vi "WRITE CAN DATA.vi"(7 "Enum":T2=enum."GET", 11 "CAN DATA":T1[](array[typedef])) -> (3 "READ DATA OUT":T1[](array[typedef]))   [LabVIEW 2025]
uses:
  Controls/READ CAN DATA.ctl
  Controls/READ CAN CLUSTER.ctl
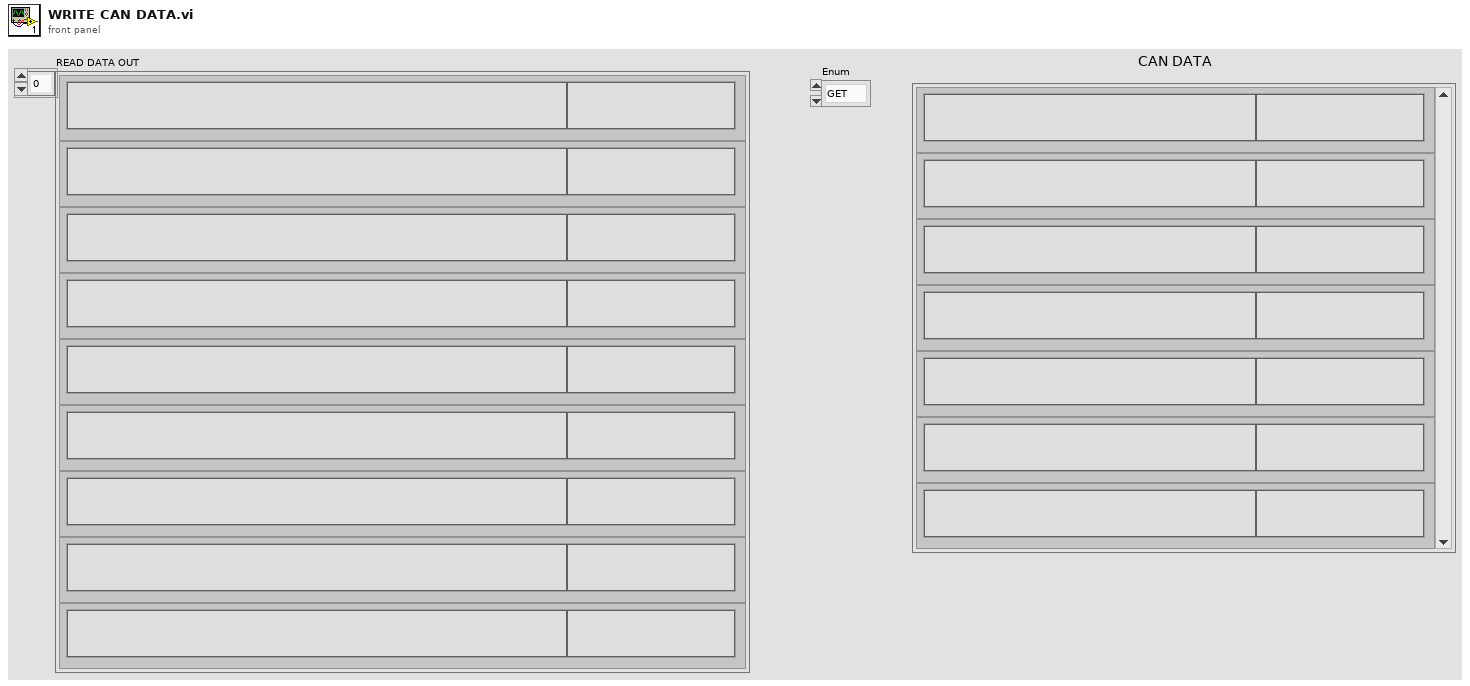
[diagram p1: front panel]
types:
  T1 = typedef "READ CAN CLUSTER.ctl" = cluster{"FUNCTION":string, "DATA":string}
  T2 = typedef "READ CAN DATA.ctl" = enum16{"SET", "GET"}
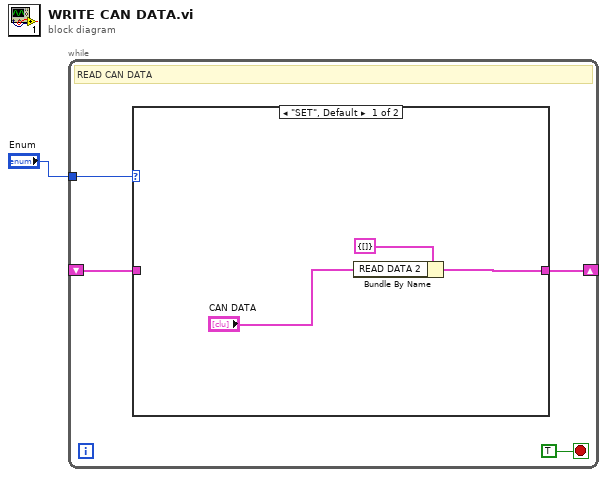
[diagram p0: block diagram]
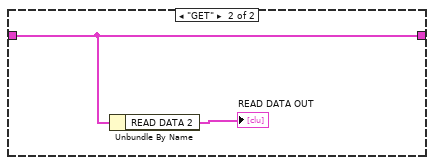
[diagram p2: hidden frame]
diagram:
  n1 = while {
    tunnel: "Enum" -> [w4]
    shift-right: [w3] -> _
    shift-left: _ -> [w2]
    stop <- TRUE stop-if-true
    # "READ CAN DATA"
    n2 = case shown="\"SET\", Default" w4 {
      tunnel: [w6 w10] -> w3
      tunnel: w2 -> [_ w10]
      frame "SET", Default {
        n3 = Bundle By Name(cluster=cluster{"READ DATA 2":T1[]} {"READ DATA 2"=[]}, "READ DATA 2"="CAN DATA") -> (w6:cluster{"READ DATA 2":T1[]})
      }
      frame "GET" {
        n4 = Unbundle By Name(w10) -> ("READ DATA 2"=→"READ DATA OUT":T1[])
      }
    }
  }
